vi "GetStatus.vi"(0 "class data in":refnum<class "AnalogComparator.lvclass">) -> (6 "Status":bool)   [LabVIEW 2019, in "AnalogComparator.lvclass"]
uses:
  AnalogComparator.lvclass
  AnalogComparator.lvclass/AnalogComparator.ctl
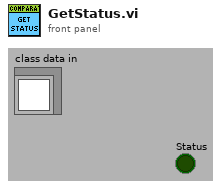
[diagram p1: front panel]
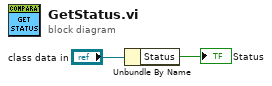
[diagram p0: block diagram]
diagram:
  n1 = Unbundle By Name("class data in") -> ("Status"=→"Status":bool)
